vi "test_emit.vi"() -> (3 "test_result":T1)   [LabVIEW 2015]
uses:
  tester_result.ctl
  result/result.lvclass/result.ctl
  input/input.lvclass
  result/result.lvclass
  output/Output.lvclass
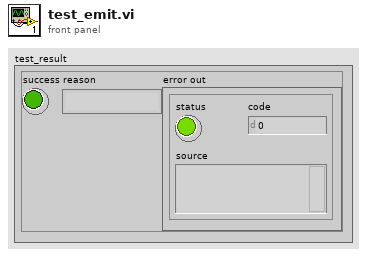
[diagram p1: front panel]
types:
  T1 = typedef "tester_result.ctl" = cluster{"success":bool, "reason":string, "error out":errorcluster}
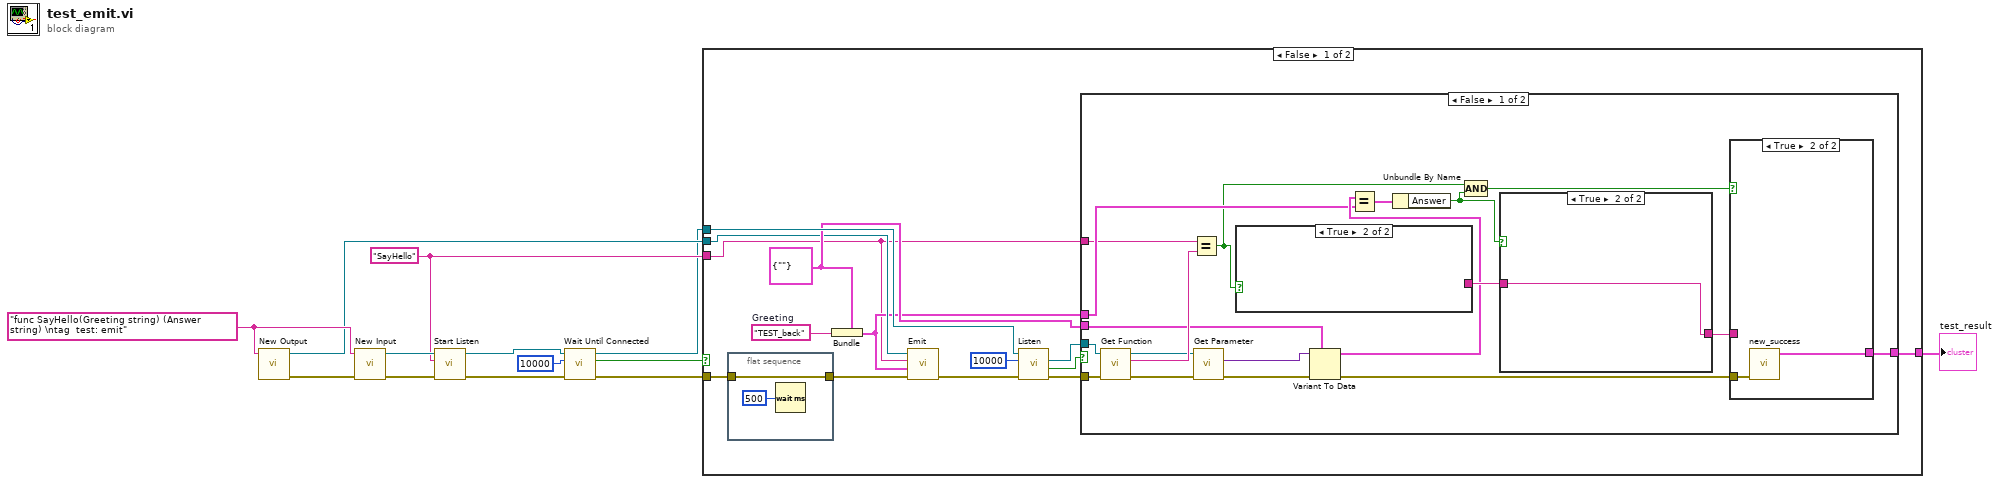
[diagram p0: block diagram]
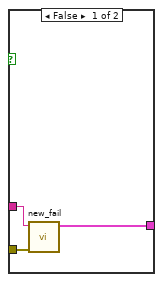
[diagram p2: hidden frame]
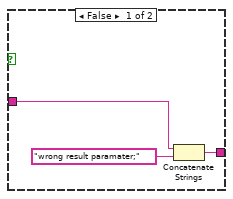
[diagram p3: hidden frame]
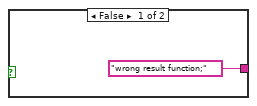
[diagram p4: hidden frame]
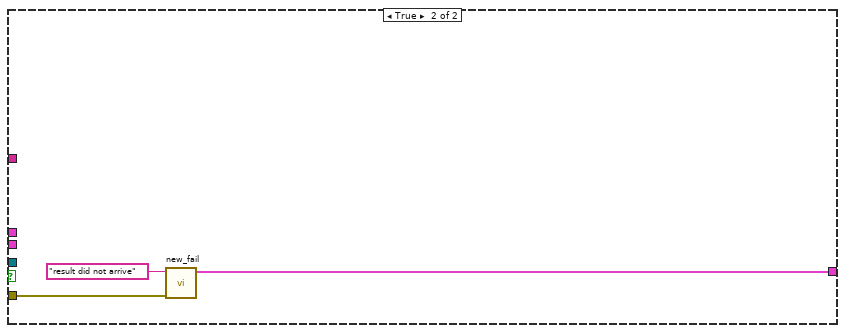
[diagram p5: hidden frame]
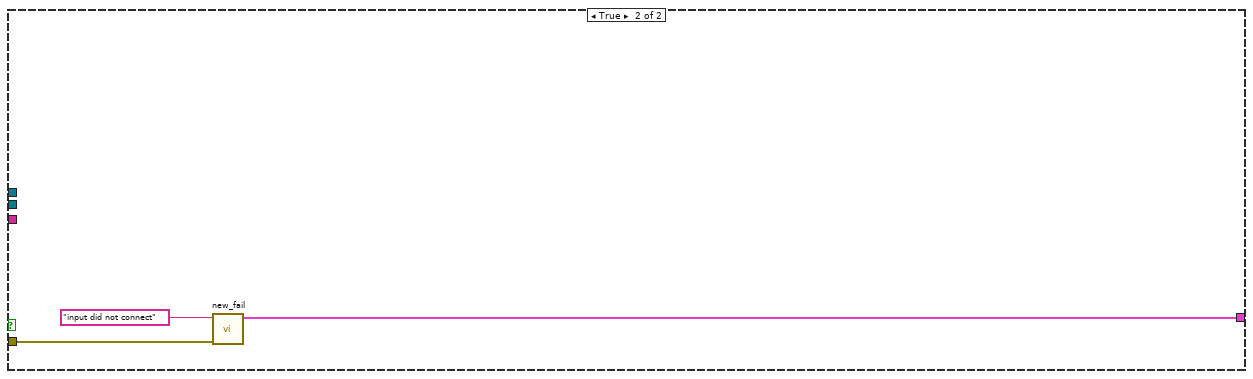
[diagram p6: hidden frame]
diagram:
  w7 = "SayHello" ("Function")
  w10 = "func SayHello(Greeting string) (Answer string) \ntag  test: emit" ("Descriptor")
  n1 = call "New Output.vi"("Descriptor"=w10) -> ("error out"=w9:errorcluster, "output"=w8:refnum<class "Output.lvclass">)  [unwired: 9 in]
  n2 = call "New Input.vi"("error in (no error)"=w9, "Descriptor"=w10) -> ("error out"=w13:errorcluster, "input out"=w12:refnum<class "input.lvclass">)  [unwired: 8 in]
  n3 = call "Start Listen.vi"("error in (no error)"=w13, "Function"=w7, "input in"=w12) -> ("error out"=w5:errorcluster, "input out"=w6:refnum<class "input.lvclass">)  [unwired: 7 in]
  n4 = call "Wait Until Connected.vi"("error in (no error)"=w5, "timeout in ms (-1)"=10000, "input in"=w6) -> ("error out"=w4:errorcluster, "timeout"=w1:bool, "input out"=w3:refnum<class "input.lvclass">)  [unwired: 6 in]
  n5 = case shown="False" w1 {
    tunnel: [w27 w62] -> w11
    tunnel: w8 -> [w19 _]
    tunnel: w7 -> [w16 _]
    tunnel: w4 -> [w14 w64]
    tunnel: w3 -> [w26 _]
    frame False {
      w25 = "TEST_back"  # Greeting
      w20 = cluster{"Answer":string} {"Answer"=""}
      n6 = flat-sequence {
        tunnel: [w29] -> w15
        tunnel: w14 -> [w29]
        frame #0 {
          n7 = Wait (ms)(milliseconds to wait=u32 500) -> ()  [unwired: 1 out]
        }
      }
      n8 = Bundle(cluster=w20, "Answer"=w25) -> (w18:cluster{"Answer":string})
      n9 = call "Emit.vi"("error in (no error)"=w15, "parameter"=w18, "function"=w16, "output in"=w19) -> ("error out"=w17:errorcluster)  [unwired: 6 in, 1 out]
      n10 = call-dynamic "Listen.vi"("error in (no error)"=w17, "timeout in ms (-1)"=10000, "input in"=w26) -> ("error out"=w24:errorcluster, "timed out?"=w22:bool, "result"=w21:refnum<class "result.lvclass">)  [unwired: 5 in, 1 out]
      n11 = case shown="False" w22 {
        tunnel: [w48 w59] -> w27
        tunnel: w24 -> [w36 w60]
        tunnel: w21 -> [w47 _]
        tunnel: w20 -> [w40 _]
        tunnel: w18 -> [w38 _]
        tunnel: w16 -> [w30 _]
        frame False {
          n12 = call "Get Function.vi"("error in (no error)"=w36, "result in"=w47) -> ("error out"=w43:errorcluster, "function"=w46:string, "result out"=w44:refnum<class "result.lvclass">)  [unwired: 7 in]
          n13 = Equal?(x=w30, y=w46) -> (x = y?=w34:bool)
          n14 = call-dynamic "Get Parameter.vi"("error in (no error)"=w43, "result in"=w44) -> ("error out"=w42:errorcluster, "Data"=w41:variant)  [unwired: 7 in, 1 out]
          n15 = case shown="True" w34 {
            tunnel: ["wrong result function;" ("source") _] -> w45
            frame False {
            }
            frame True {
            }
          }
          n16 = Variant To Data(error in=w42, type=w40, Variant=w41) -> (data=w39:cluster{"Answer":string}, error out=w35:errorcluster)
          n17 = Equal?(x=w39, y=w38) -> (x = y?=w37:cluster{"Answer":bool})
          n18 = Unbundle By Name(w37) -> ("Answer"=w31:bool)
          n19 = Compound Arithmetic op=AND(w34, w31) -> (w33:bool)
          n20 = case shown="True" w31 {
            tunnel: w45 -> [w56 w57]
            tunnel: [w54 w57] -> w32
            frame False {
              n21 = Concatenate Strings(w56, "wrong result paramater;" ("source")) -> (w54:string)
            }
            frame True {
            }
          }
          n22 = case shown="True" w33 {
            tunnel: [w49 w52] -> w48
            tunnel: w35 -> [w50 w53]
            tunnel: w32 -> [w51 _]
            frame False {
              n23 = call "new_fail.vi"("error out"=w50, "reason"=w51) -> ("result"=w49:T1)  [unwired: 9 in]
            }
            frame True {
              n24 = call "new_success.vi"("error out"=w53) -> ("result"=w52:T1)  [unwired: 10 in]
            }
          }
        }
        frame True {
          n25 = call "new_fail.vi"("error out"=w60, "reason"="result did not arrive") -> ("result"=w59:T1)  [unwired: 9 in]
        }
      }
    }
    frame True {
      n26 = call "new_fail.vi"("error out"=w64, "reason"="input did not connect") -> ("result"=w62:T1)  [unwired: 9 in]
    }
  }
  "test_result" <- w11
